vi "Parse Control Data Z.vi"(0 "control type":u16, 1 "offset":i32, 2 "cluster data":string, 3 "error in":T1, 4 "floating-point type conversion":string[][](table)=[["extended", "5", "12"], ["double", "5", "9"], ["single", "5", "5"]]) -> (5 "data value":string, 6 "offset past cluster data":i32, 7 "error out":T1)   [LabVIEW 2016]
doc: "Determines a cluster's data values from the flattened cluster.\nModified from the original SQL add-on version, to save floating-point numbers in exponential format. The only change is the use of the \"To Exponential\" function in place of \"To Fractional\""
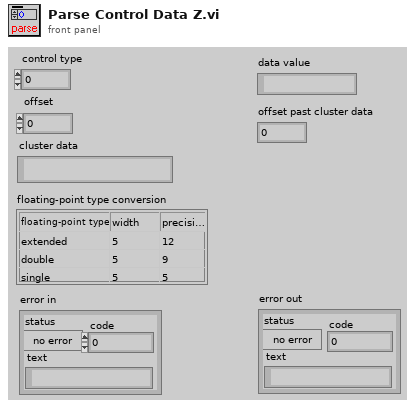
[diagram p1: front panel]
types:
  T1 = cluster{"status":bool, "code":i32, "text":string}
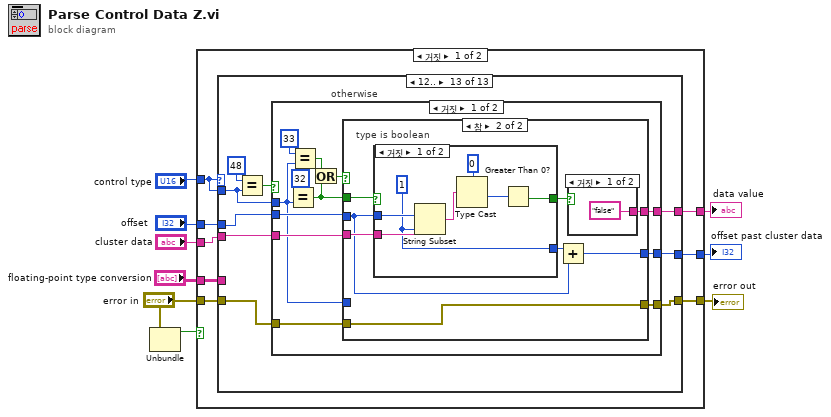
[diagram p0: block diagram]
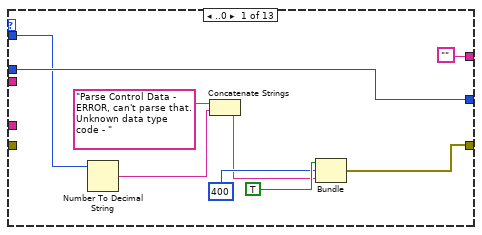
[diagram p2: hidden frame]
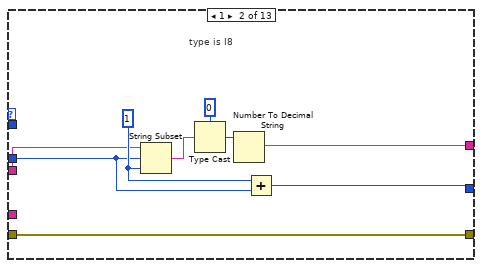
[diagram p3: hidden frame]
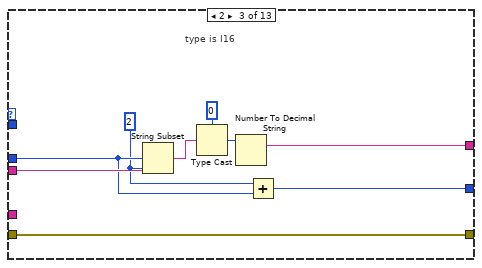
[diagram p4: hidden frame]
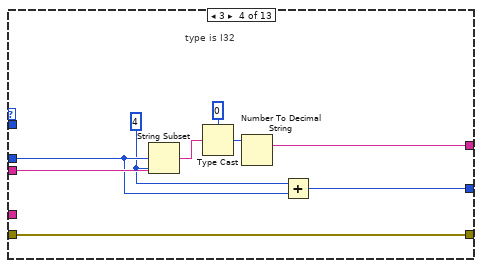
[diagram p5: hidden frame]
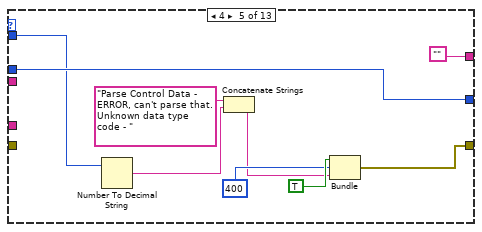
[diagram p6: hidden frame]
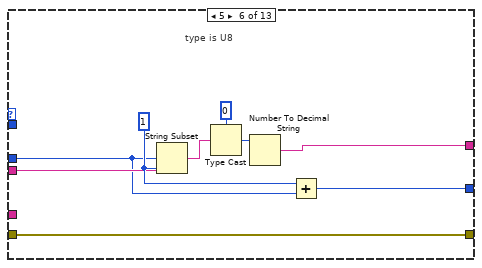
[diagram p7: hidden frame]
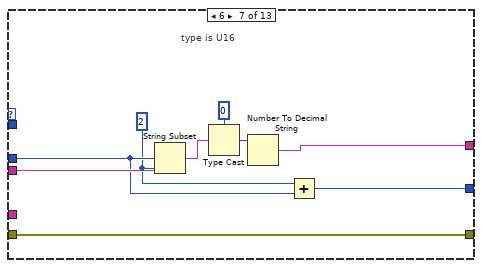
[diagram p8: hidden frame]
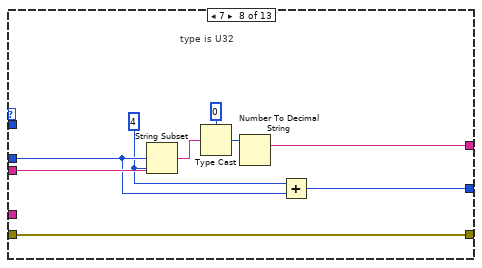
[diagram p9: hidden frame]
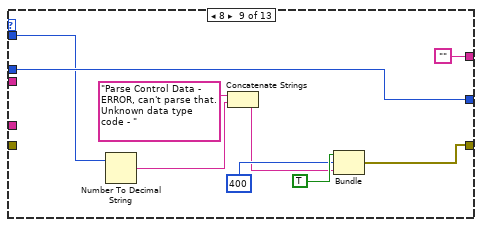
[diagram p10: hidden frame]
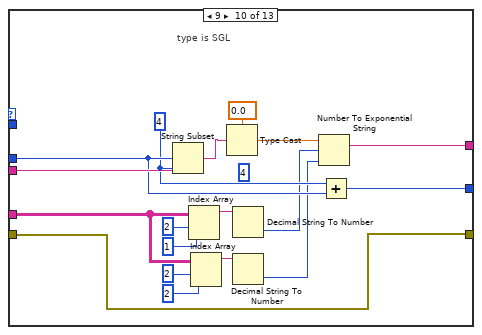
[diagram p11: hidden frame]
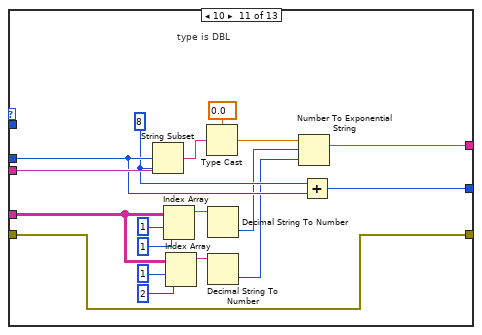
[diagram p12: hidden frame]
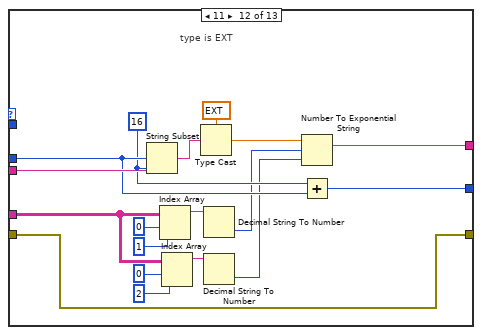
[diagram p13: hidden frame]
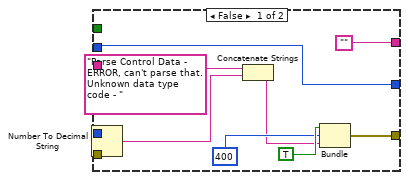
[diagram p14: hidden frame]
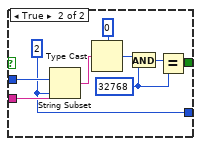
[diagram p15: hidden frame]
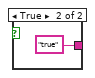
[diagram p16: hidden frame]
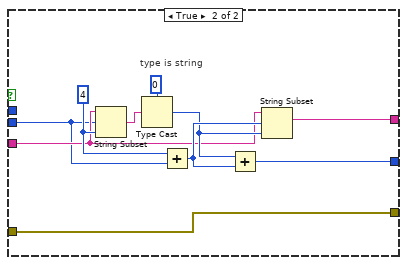
[diagram p17: hidden frame]
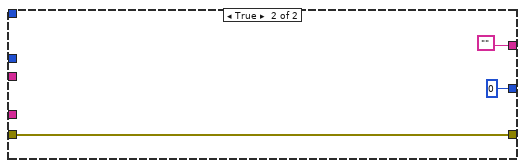
[diagram p18: hidden frame]
diagram:
  n1 = Unbundle("error in") -> ("status"=w4:bool)  [unwired: 2 out]
  n2 = case shown="거짓" w4 {
    tunnel: "control type" -> [w17 _]
    tunnel: "offset" -> [w16 _]
    tunnel: "cluster data" -> [w15 _]
    tunnel: "floating-point type conversion" -> [w14 _]
    tunnel: [w10 w221] -> w3
    tunnel: "error in" -> [w11 w221]
    tunnel: [w13 0] -> w2
    tunnel: [w12 ""] -> w1
    frame False {
      n3 = case shown="12.." w17 {
        tunnel: w15 -> [_ w31 w44 w53 _ w67 w80 w89 _ w116 w134 w152 w159]
        tunnel: w16 -> [w26 w30 w42 w51 w62 w66 w78 w87 w98 w114 w132 w150 w158]
        tunnel: [w26 w29 w40 w49 w62 w65 w76 w85 w98 w109 w128 w146 w157] -> w13
        tunnel: ["" w28 w37 w46 "" w64 w73 w82 "" w112 w130 w148 w156] -> w12
        tunnel: w14 -> [_ _ _ _ _ _ _ _ _ w100 w119 w137 _]
        tunnel: w17 -> [w18 _ _ _ w55 _ _ _ w91 _ _ _ w155]
        tunnel: w11 -> [_ w27 w36 w45 _ w63 w72 w81 _ w99 w117 w135 w153]
        tunnel: [w20 w27 w36 w45 w56 w63 w72 w81 w92 w99 w117 w135 w154] -> w10
        frame ..0 {
          n4 = Number To Decimal String(number=w18) -> (decimal integer string=w22:string)  [unwired: 1 in]
          n5 = Concatenate Strings("Parse Control Data - ERROR, can't parse that.  Unknown data type code - ", w22) -> (w21:string)
          n6 = Bundle(TRUE, 400, w21) -> (w20:errorcluster)  [unwired: 1 in]
        }
        frame 1 {
          w34 = 1
          # "type is I8"
          n7 = String Subset(string=w31, offset (0)=w30, length (rest)=w34) -> (substring=w33:string)
          n8 = Type Cast(type=i8 0, x=w33) -> (*(type *) &x=w32:i8)
          n9 = Number To Decimal String(number=w32) -> (decimal integer string=w28:string)  [unwired: 1 in]
          n10 = Add(x=w34, y=w30) -> (x+y=w29:i32)
        }
        frame 2 {
          w41 = 2
          # "type is I16"
          n11 = String Subset(string=w44, offset (0)=w42, length (rest)=w41) -> (substring=w39:string)
          n12 = Type Cast(type=i16 0, x=w39) -> (*(type *) &x=w38:i16)
          n13 = Number To Decimal String(number=w38) -> (decimal integer string=w37:string)  [unwired: 1 in]
          n14 = Add(x=w41, y=w42) -> (x+y=w40:i32)
        }
        frame 3 {
          w50 = 4
          # "type is I32"
          n15 = String Subset(string=w53, offset (0)=w51, length (rest)=w50) -> (substring=w48:string)
          n16 = Type Cast(type=0, x=w48) -> (*(type *) &x=w47:i32)
          n17 = Number To Decimal String(number=w47) -> (decimal integer string=w46:string)  [unwired: 1 in]
          n18 = Add(x=w50, y=w51) -> (x+y=w49:i32)
        }
        frame 4 {
          n19 = Number To Decimal String(number=w55) -> (decimal integer string=w58:string)  [unwired: 1 in]
          n20 = Concatenate Strings("Parse Control Data - ERROR, can't parse that.  Unknown data type code - ", w58) -> (w57:string)
          n21 = Bundle(TRUE, 400, w57) -> (w56:errorcluster)  [unwired: 1 in]
        }
        frame 5 {
          w70 = 1
          # "type is U8"
          n22 = String Subset(string=w67, offset (0)=w66, length (rest)=w70) -> (substring=w69:string)
          n23 = Type Cast(type=u8 0, x=w69) -> (*(type *) &x=w68:u8)
          n24 = Number To Decimal String(number=w68) -> (decimal integer string=w64:string)  [unwired: 1 in]
          n25 = Add(x=w70, y=w66) -> (x+y=w65:i32)
        }
        frame 6 {
          w77 = 2
          # "type is U16"
          n26 = String Subset(string=w80, offset (0)=w78, length (rest)=w77) -> (substring=w75:string)
          n27 = Type Cast(type=u16 0, x=w75) -> (*(type *) &x=w74:u16)
          n28 = Number To Decimal String(number=w74) -> (decimal integer string=w73:string)  [unwired: 1 in]
          n29 = Add(x=w77, y=w78) -> (x+y=w76:i32)
        }
        frame 7 {
          w86 = 4
          # "type is U32"
          n30 = String Subset(string=w89, offset (0)=w87, length (rest)=w86) -> (substring=w84:string)
          n31 = Type Cast(type=u32 0, x=w84) -> (*(type *) &x=w83:u32)
          n32 = Number To Decimal String(number=w83) -> (decimal integer string=w82:string)  [unwired: 1 in]
          n33 = Add(x=w86, y=w87) -> (x+y=w85:i32)
        }
        frame 8 {
          n34 = Number To Decimal String(number=w91) -> (decimal integer string=w94:string)  [unwired: 1 in]
          n35 = Concatenate Strings("Parse Control Data - ERROR, can't parse that.  Unknown data type code - ", w94) -> (w93:string)
          n36 = Bundle(TRUE, 400, w93) -> (w92:errorcluster)  [unwired: 1 in]
        }
        frame 9 {
          (unwired) 4
          w110 = 4
          # "type is SGL"
          n37 = String Subset(string=w116, offset (0)=w114, length (rest)=w110) -> (substring=w111:string)
          n38 = Index Array(array=w100, index (row)=2, index (col)=1) -> (element=w106:string)
          n39 = Index Array(array=w100, index (row)=2, index (col)=2) -> (element=w102:string)
          n40 = Type Cast(type=sgl 0.0, x=w111) -> (*(type *) &x=w113:sgl)
          n41 = Decimal String To Number(string=w106) -> (number=w105:i32)  [unwired: 2 in, 1 out]
          n42 = Decimal String To Number(string=w102) -> (number=w101:i32)  [unwired: 2 in, 1 out]
          n43 = Number To Exponential String(number=w113, precision (6)=w101, 3:w105) -> (E-format string=w112:string)  [unwired: 1 in]
          n44 = Add(x=w110, y=w114) -> (x+y=w109:i32)
        }
        frame 10 {
          w131 = 8
          # "type is DBL"
          n45 = String Subset(string=w134, offset (0)=w132, length (rest)=w131) -> (substring=w127:string)
          n46 = Index Array(array=w119, index (row)=1, index (col)=1) -> (element=w124:string)
          n47 = Index Array(array=w119, index (row)=1, index (col)=2) -> (element=w122:string)
          n48 = Type Cast(type=0.0, x=w127) -> (*(type *) &x=w129:dbl)
          n49 = Decimal String To Number(string=w124) -> (number=w121:i32)  [unwired: 2 in, 1 out]
          n50 = Decimal String To Number(string=w122) -> (number=w120:i32)  [unwired: 2 in, 1 out]
          n51 = Number To Exponential String(number=w129, precision (6)=w120, 3:w121) -> (E-format string=w130:string)  [unwired: 1 in]
          n52 = Add(x=w131, y=w132) -> (x+y=w128:i32)
        }
        frame 11 {
          w149 = 16
          # "type is EXT"
          n53 = String Subset(string=w152, offset (0)=w150, length (rest)=w149) -> (substring=w145:string)
          n54 = Index Array(array=w137, index (row)=0, index (col)=1) -> (element=w142:string)
          n55 = Index Array(array=w137, index (row)=0, index (col)=2) -> (element=w140:string)
          n56 = Type Cast(type=ext 0.0, x=w145) -> (*(type *) &x=w147:ext)
          n57 = Decimal String To Number(string=w142) -> (number=w139:i32)  [unwired: 2 in, 1 out]
          n58 = Decimal String To Number(string=w140) -> (number=w138:i32)  [unwired: 2 in, 1 out]
          n59 = Number To Exponential String(number=w147, precision (6)=w138, 3:w139) -> (E-format string=w148:string)  [unwired: 1 in]
          n60 = Add(x=w149, y=w150) -> (x+y=w146:i32)
        }
        frame 12.. {
          # "otherwise"
          n61 = Equal?(x=48, y=w155) -> (x = y?=w160:bool)
          n62 = case shown="거짓" w160 {
            tunnel: w159 -> [w172 w213]
            tunnel: w158 -> [w171 w212]
            tunnel: [w169 w211] -> w157
            tunnel: [w170 w210] -> w156
            tunnel: w155 -> [w166 _]
            tunnel: [w168 w209] -> w154
            tunnel: w153 -> [w167 w209]
            frame False {
              n63 = Equal?(x=32, y=w166) -> (x = y?=w162:bool)
              n64 = Equal?(x=33, y=w166) -> (x = y?=w164:bool)
              n65 = Or(x=w164, y=w162) -> (x .or. y?=w163:bool)
              n66 = case shown="참" w163 {
                tunnel: w172 -> [_ w189]
                tunnel: w171 -> [w181 w188]
                tunnel: ["" w187] -> w170
                tunnel: [w181 w186] -> w169
                tunnel: [w180 w185] -> w168
                tunnel: w166 -> [w177 _]
                tunnel: w167 -> [_ w185]
                tunnel: w162 -> [_ w184]
                frame False {
                  n67 = Number To Decimal String(number=w177) -> (decimal integer string=w175:string)  [unwired: 1 in]
                  n68 = Concatenate Strings("Parse Control Data - ERROR, can't parse that.  Unknown data type code - ", w175) -> (w174:string)
                  n69 = Bundle(TRUE, 400, w174) -> (w180:errorcluster)  [unwired: 1 in]
                }
                frame True {
                  # "type is boolean"
                  n70 = case shown="거짓" w184 {
                    tunnel: w188 -> [w195 w203]
                    tunnel: w189 -> [w194 w202]
                    tunnel: [w193 w201] -> w190
                    tunnel: [w192 w198] -> w183
                    frame False {
                      w193 = 1
                      n71 = String Subset(string=w194, offset (0)=w195, length (rest)=w193) -> (substring=w197:string)
                      n72 = Type Cast(type=u8 0, x=w197) -> (*(type *) &x=w191:u8)
                      n73 = Greater Than 0?(x=w191) -> (x > 0?=w192:bool)
                    }
                    frame True {
                      w200 = u16 32768
                      w201 = 2
                      n74 = String Subset(string=w202, offset (0)=w203, length (rest)=w201) -> (substring=w205:string)
                      n75 = Type Cast(type=u16 0, x=w205) -> (*(type *) &x=w206:u16)
                      n76 = And(x=w206, y=w200) -> (x .and. y?=w199:u16)
                      n77 = Equal?(x=w199, y=w200) -> (x = y?=w198:bool)
                    }
                  }
                  n78 = Add(x=w190, y=w188) -> (x+y=w186:i32)
                  n79 = case shown="거짓" w183 {
                    tunnel: ["false" "true"] -> w187
                    frame False {
                    }
                    frame True {
                    }
                  }
                }
              }
            }
            frame True {
              w216 = 4
              # "type is string"
              n80 = String Subset(string=w213, offset (0)=w212, length (rest)=w216) -> (substring=w218:string)
              n81 = Type Cast(type=0, x=w218) -> (*(type *) &x=w214:i32)
              n82 = Add(x=w216, y=w212) -> (x+y=w215:i32)
              n83 = Add(x=w214, y=w215) -> (x+y=w211:i32)
              n84 = String Subset(string=w213, offset (0)=w215, length (rest)=w214) -> (substring=w210:string)
            }
          }
        }
      }
    }
    frame True {
    }
  }
  "offset past cluster data" <- w2
  "data value" <- w1
  "error out" <- w3
